vi "Read experiment parameter.vi"(8 "error in":errorcluster, 9 "Exp. file path":path, 10 "Reaction parameter in":T1={"Pump 1 refill rate (ml/min) "=6.0, "Pump 1 refill volume (mL)"=1.8, "Pump 1 transfer rate (ml/min)"=0.08, "Pump 1 oscill. rate (ml/min)"=0.04, "Vertex potential 1(V)"=-0.5, "Initial potential (V)"=0.0, "Final potential (V)"=0.0, "Cycles"=1, "Delayed time for waiting(s)"=5.0, "Pressure (psi)"=15.0, "Vertex potential 2(V)"=0.0, "Use inital potential?"=TRUE, "Sample name"="", "To waste flow factor"=5.0, "Temperature (C)"=20.0, "Scan rate (V/s)"=10.0, "Use final potential?"=TRUE, "CV current range"="20MA", "Cell to use"="EXTERNAL"} {"Scan rate (V/s)" min=0.0 max=10.0 format="%#_4f"; "Vertex potential 2(V)" min=-5.0 max=5.0 format="%.3f"; "Cycles" min=1 max=30; "Final potential (V)" min=-5.0 format="%_3f"; "Initial potential (V)" min=-5.0 max=5.0 format="%.3f"; "Vertex potential 1(V)" min=-5.0 max=5.0 format="%.3f"; "Pump 1 oscill. rate (ml/min)" format="%#.4f"; "Pump 1 transfer rate (ml/min)" format="%#.4f"; "Pump 1 refill volume (mL)" format="%#.4f"; "Pump 1 refill rate (ml/min)" format="%#.4f"}, 11 "ALS mode parameter in":T2={"Wash vial Location"=0.0, "Reagent volume (ul)"=[], "Reagent location"=[], "Mix vial Location"=0.0, "Pump 5 target volume (ml)"=5.0, "Pump 5  flowrate (ml/min)"=5.0, "Sample name"=""} {"Pump 5  flowrate (ml/min)" min=0.0 format="%#.4f"; "Pump 5 target volume (ml)" min=0.0 format="%#.4f"}) -> (0 "error out":errorcluster, 1 "expInfo":string, 2 "Reaction parameter out":T1={"Pump 1 refill rate (ml/min) "=6.0, "Pump 1 refill volume (mL)"=1.8, "Pump 1 transfer rate (ml/min)"=0.08, "Pump 1 oscill. rate (ml/min)"=0.04, "Vertex potential 1(V)"=-0.5, "Initial potential (V)"=0.0, "Final potential (V)"=0.0, "Cycles"=1, "Delayed time for waiting(s)"=5.0, "Pressure (psi)"=15.0, "Vertex potential 2(V)"=0.0, "Use inital potential?"=TRUE, "Sample name"="", "To waste flow factor"=5.0, "Temperature (C)"=20.0, "Scan rate (V/s)"=10.0, "Use final potential?"=TRUE, "CV current range"="20MA", "Cell to use"="EXTERNAL"} {"Scan rate (V/s)" min=0.0 max=10.0 format="%#_4f"; "Vertex potential 2(V)" min=-5.0 max=5.0 format="%.3f"; "Cycles" min=1 max=30; "Final potential (V)" min=-5.0 format="%_3f"; "Initial potential (V)" min=-5.0 max=5.0 format="%.3f"; "Vertex potential 1(V)" min=-5.0 max=5.0 format="%.3f"; "Pump 1 oscill. rate (ml/min)" format="%#.4f"; "Pump 1 transfer rate (ml/min)" format="%#.4f"; "Pump 1 refill volume (mL)" format="%#.4f"; "Pump 1 refill rate (ml/min)" format="%#.4f"}, 3 "ALS mode parameter out":T2={"Wash vial Location"=0.0, "Reagent volume (ul)"=[], "Reagent location"=[], "Mix vial Location"=0.0, "Pump 5 target volume (ml)"=5.0, "Pump 5  flowrate (ml/min)"=5.0, "Sample name"=""} {"Pump 5  flowrate (ml/min)" min=0.0 format="%#.4f"; "Pump 5 target volume (ml)" min=0.0 format="%#.4f"}, 4 "Finished?":bool, 5 "Index":i32)   [LabVIEW 2017]
panel:
  # "Indicate whether to run."
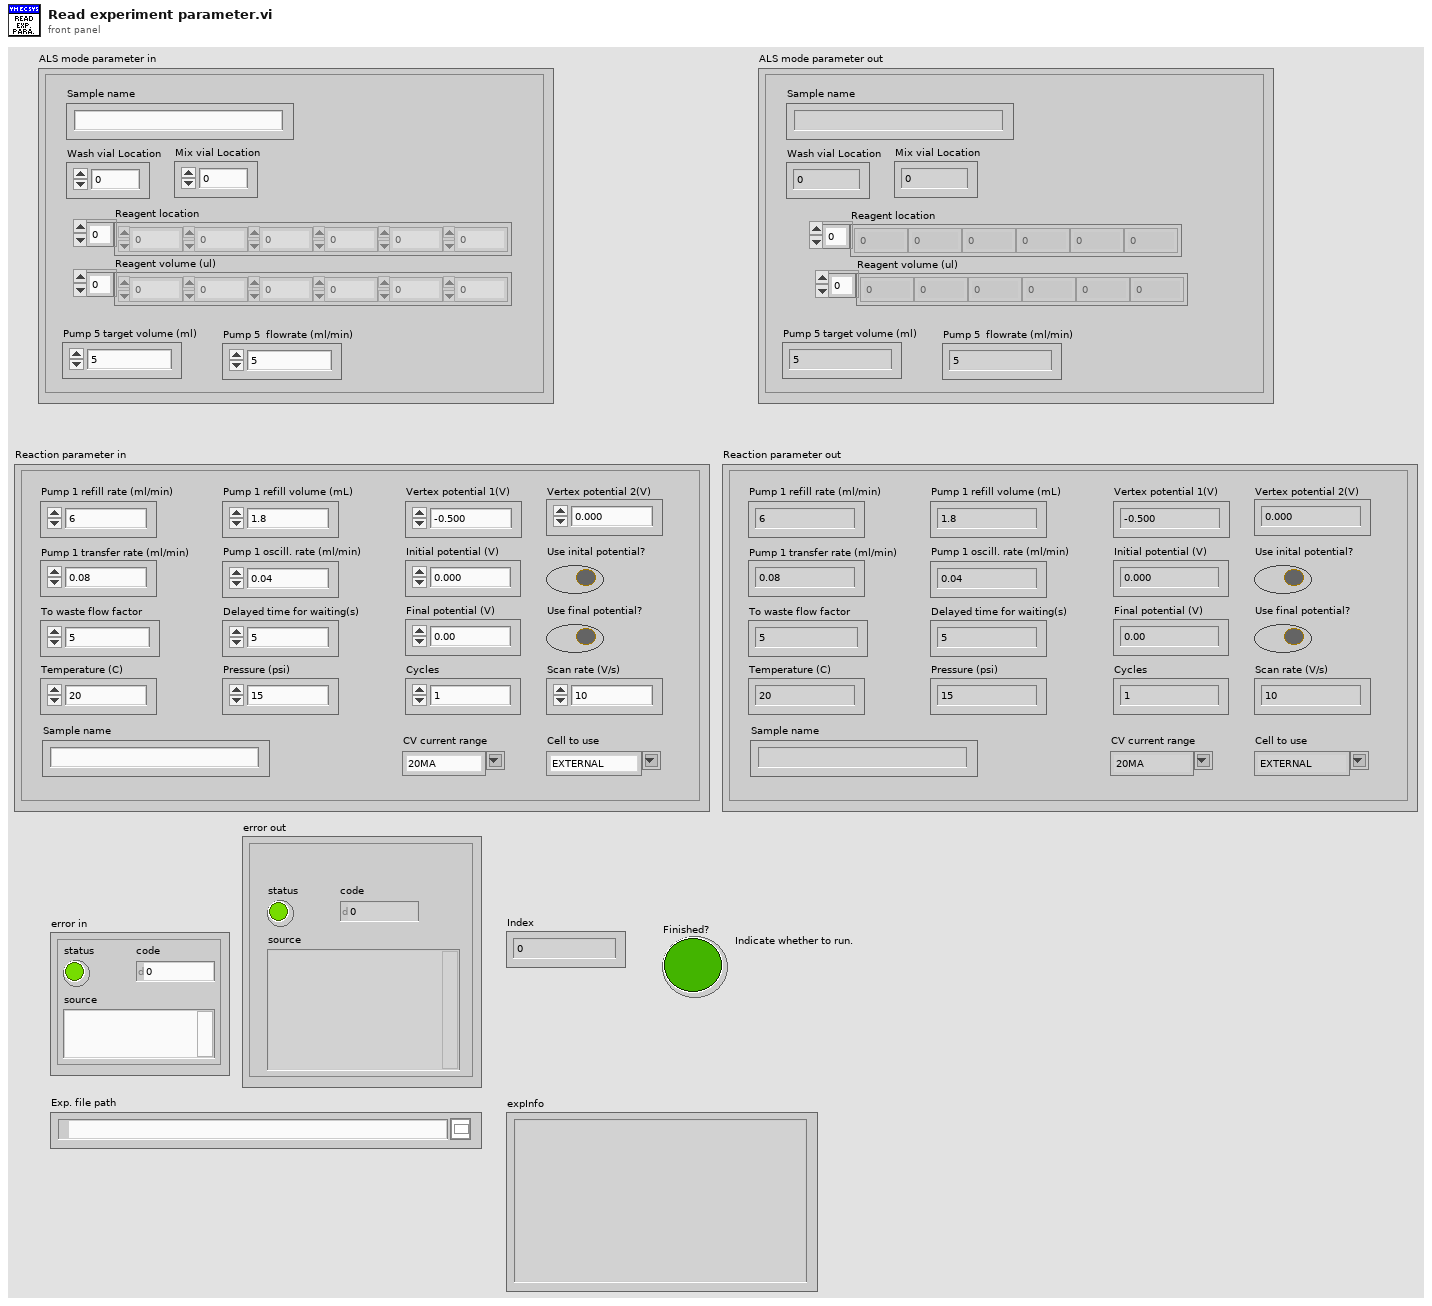
[diagram p1: front panel]
types:
  T1 = cluster{"Pump 1 refill rate (ml/min) ":dbl, "Pump 1 refill volume (mL)":dbl, "Pump 1 transfer rate (ml/min)":dbl, "Pump 1 oscill. rate (ml/min)":dbl, "Vertex potential 1(V)":dbl, "Initial potential (V)":dbl, "Final potential (V)":dbl, "Cycles":i32, "Delayed time for waiting(s)":dbl, "Pressure (psi)":dbl, "Vertex potential 2(V)":dbl, "Use inital potential?":bool, "Sample name":string, "To waste flow factor":dbl, "Temperature (C)":dbl, "Scan rate (V/s)":dbl, "Use final potential?":bool, "CV current range":string, "Cell to use":string}
  T2 = cluster{"Wash vial Location":dbl, "Reagent volume (ul)":dbl[], "Reagent location":dbl[], "Mix vial Location":dbl, "Pump 5 target volume (ml)":dbl, "Pump 5  flowrate (ml/min)":dbl, "Sample name":string}
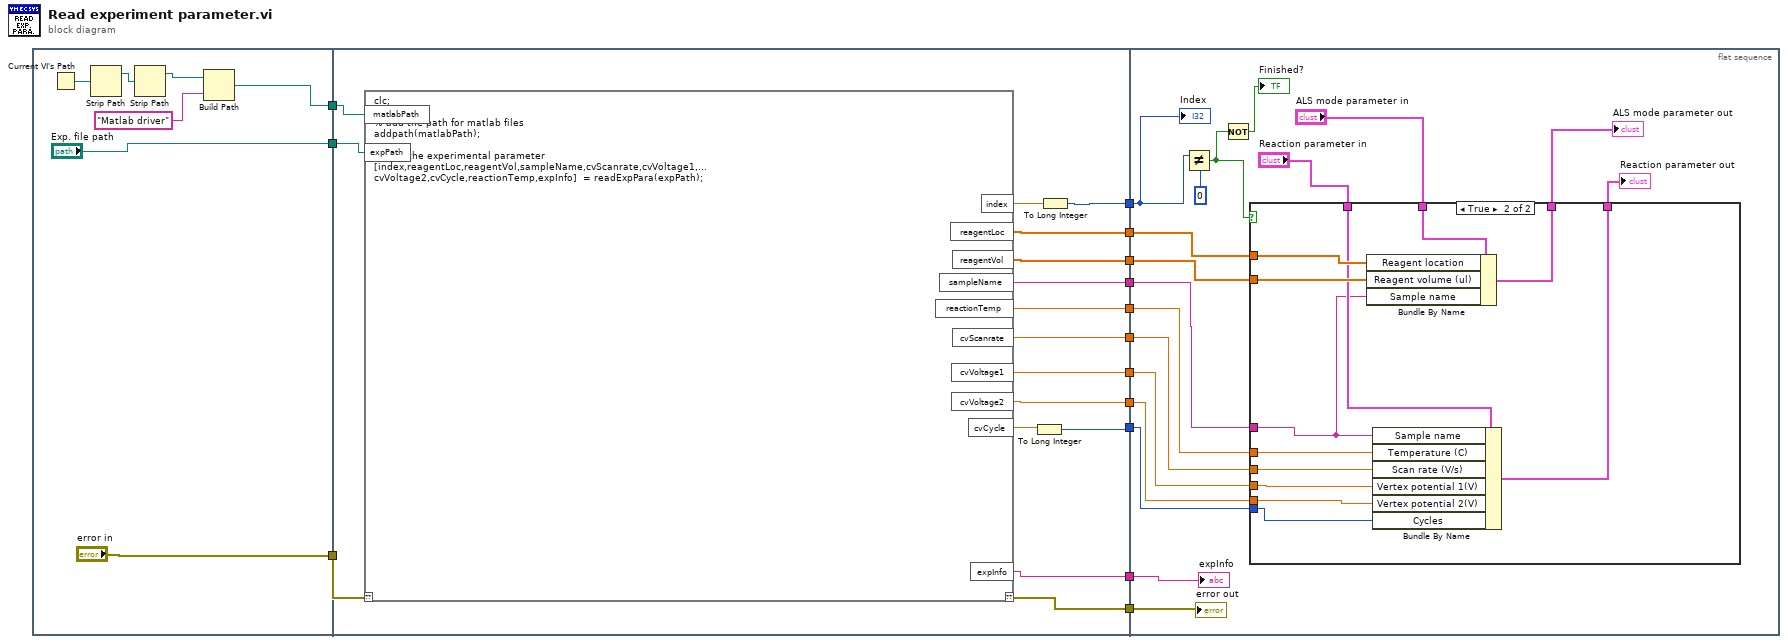
[diagram p0: block diagram]
diagram:
  n1 = flat-sequence {
    tunnel: [w17] -> w14
    tunnel: ["error in"] -> w13
    tunnel: ["Exp. file path"] -> w12
    tunnel: w14 -> [w37]
    tunnel: w13 -> [w34]
    tunnel: w12 -> [w36]
    tunnel: [w35] -> w11
    tunnel: [w33] -> w10
    tunnel: [w24] -> w9
    tunnel: [w23] -> w8
    tunnel: [w32] -> w7
    tunnel: [w31] -> w6
    tunnel: [w30] -> w5
    tunnel: [w29] -> w4
    tunnel: [w28] -> w3
    tunnel: [w27] -> w2
    tunnel: [w26] -> w1
    tunnel: w11 -> [w55]
    tunnel: w10 -> [w54]
    tunnel: w9 -> [w53]
    tunnel: w8 -> [w52]
    tunnel: w7 -> [w51]
    tunnel: w6 -> [w50]
    tunnel: w5 -> [w49]
    tunnel: w4 -> [w48]
    tunnel: w3 -> [w38]
    tunnel: w2 -> [w47]
    tunnel: w1 -> [w46]
    frame #0 {
      n2 = Current VI's Path() -> (path=w21:path)
      n3 = Strip Path(path=w21) -> (stripped path=w19:path)  [unwired: 1 out]
      n4 = Strip Path(path=w19) -> (stripped path=w18:path)  [unwired: 1 out]
      n5 = Build Path(base path=w18, name or relative path="Matlab driver") -> (appended path=w17:path)
    }
    frame #1 {
      n6 = script code="clc;\n\n% add the path for matlab files\naddpath(matlabPath);\n\n%read the experimental parameter\n[index,reagentLoc,reagentVol,sampleName,cvScanrate,cvVoltage1,...\ncvVoltage2,cvCycle,reactionTemp,expInfo]  = readExpPara(expPath);"("??"=w34, "matlabPath"=w37, "expPath"=w36) -> ("??"=w33:errorcluster, "index"=w25:dbl, "reagentLoc"=w27:dbl[], "reagentVol"=w26:dbl[], "reactionTemp"=w29:dbl, "cvScanrate"=w30:dbl, "cvVoltage1"=w31:dbl, "cvVoltage2"=w32:dbl, "cvCycle"=w22:dbl, "sampleName"=w28:string, "expInfo"=w35:string)
      n7 = To Long Integer(number=w22) -> (32bit integer=w23:i32)
      n8 = To Long Integer(number=w25) -> (32bit integer=w24:i32)
    }
    frame #2 {
      n9 = Not Equal?(x=w53, y=0) -> (x != y?=w43:bool)
      n10 = Not(x=w43) -> (.not. x?=→"Finished?":bool)
      n11 = case shown="True" w43 {
        tunnel: w52 -> [_ w58]
        tunnel: w51 -> [_ w69]
        tunnel: w50 -> [_ w68]
        tunnel: w49 -> [_ w67]
        tunnel: w48 -> [_ w66]
        tunnel: w38 -> [_ w59]
        tunnel: w47 -> [_ w65]
        tunnel: w46 -> [_ w64]
        tunnel: [w57 w63] -> w45
        tunnel: [w56 w62] -> w39
        tunnel: "ALS mode parameter in" -> [w57 w61]
        tunnel: "Reaction parameter in" -> [w56 w60]
        frame False {
        }
        frame True {
          n12 = Bundle By Name(cluster=w61, "Reagent location"=w65, "Reagent volume (ul)"=w64, "Sample name"=w59) -> (w63:T2)
          n13 = Bundle By Name(cluster=w60, "Sample name"=w59, "Temperature (C)"=w66, "Scan rate (V/s)"=w67, "Vertex potential 1(V)"=w68, "Vertex potential 2(V)"=w69, "Cycles"=w58) -> (w62:T1)
        }
      }
      "ALS mode parameter out" <- w45
      "Reaction parameter out" <- w39
      "expInfo" <- w55
      "error out" <- w54
      "Index" <- w53
    }
  }
